vi "PLF.vi"(5 "ActivateAIView":bool, 9 "curr_pos":dbl=50.0 min=50.0 max=150.0, 10 "Y":refnum<data-value>, 11 "K":refnum<data-value>) -> (3 "This VI":refnum<vi>)   [LabVIEW 2019]
uses:
  Inputs/Inputs.lvlib
panel:
  in  "обнулить позицию":bool
  in  "pos_offset":dbl=50.0 min=2.0 max=120.0
  in  "зона нечувствительности":dbl
  in  "Q in":dbl format="%#.2f"
  out "Y 2":dbl format="%#.2f"
  out "XY Graph":cluster{"SP_massiv":dbl[], "Y_massiv":dbl[]}(graph)
  in  "Y_massiv":dbl[](array[numeric]) format="%#.2f"
  in  "SP_massiv":dbl[](array[numeric]) format="%#.2f"
  in  "derivative time (Td, s)":dbl
  in  "integral time (Ti, s)":dbl
  in  "proportional gain (Kc)":dbl
  in  "output high":dbl
  # "Параметры ПИД Регулятора"
  # "Y"
  # "Настройка Выхода"
  # "Q_max"
  # "Q9"
  # "Q8"
  # "Q7"
  # "Q6"
  # "Q5"
  # "Q4"
  # "Q3"
  # "Q2"
  # "Q1"
  # "Q_min"
  # "X"
  # "Y_min"
  # "Y1"
  # "Y2"
  # "Y3"
  # "Y4"
  # "Y5"
  # "Y6"
  # "Y7"
  # "Y8"
  # "Y9"
  # "Y_max"
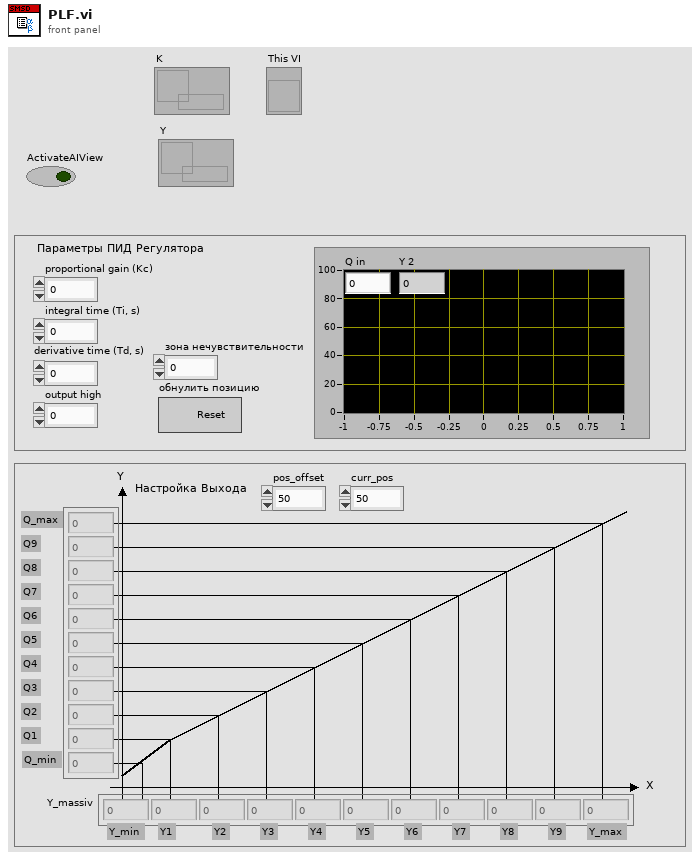
[diagram p1: front panel]
types:
  T1 = enum32{"Invalid", "Standard", "Closed", "Hidden", "Minimized", "Maximized"}
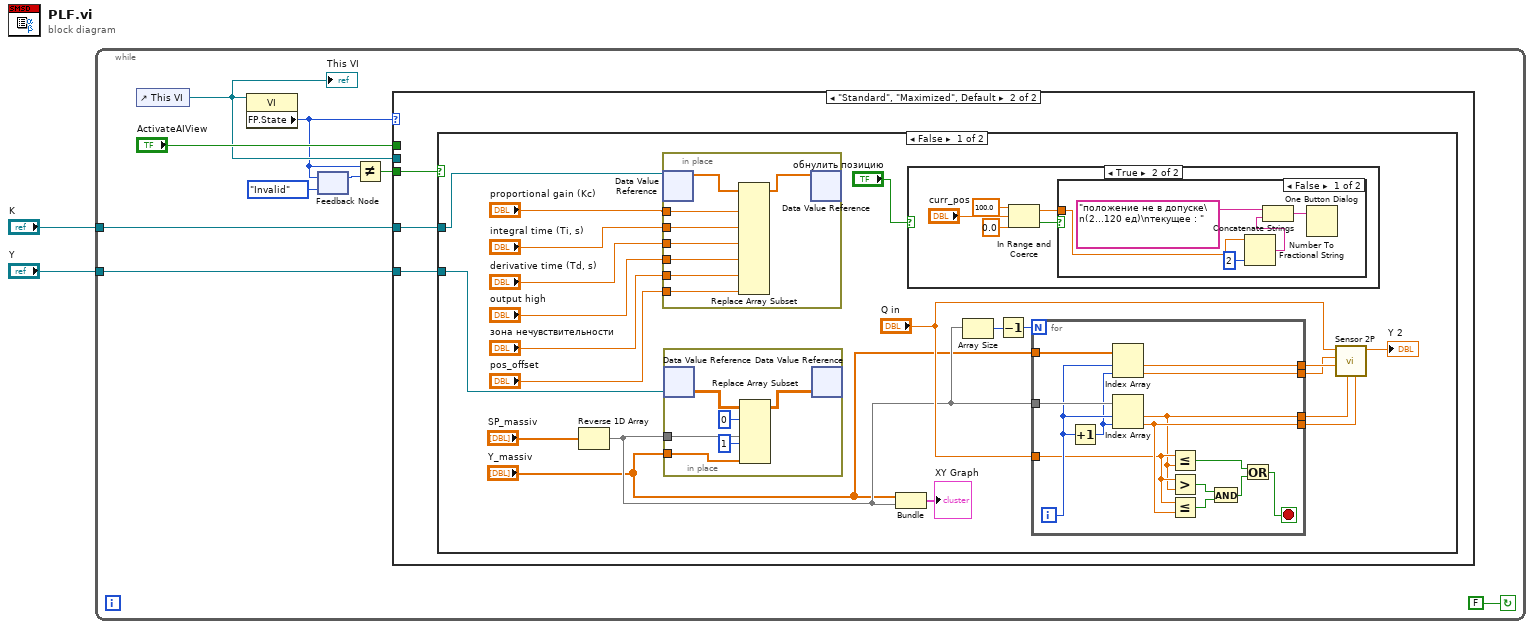
[diagram p0: block diagram]
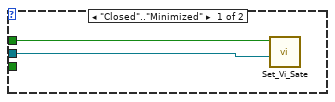
[diagram p2: hidden frame]
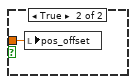
[diagram p4: hidden frame]
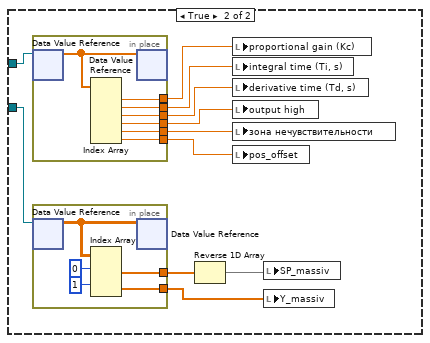
[diagram p5: hidden frame]
diagram:
  n1 = while {
    tunnel: "K" -> [w4]
    tunnel: "Y" -> [w3]
    stop <- FALSE continue-if-true
    n2 = control-ref of="This VI"() -> (w10:refnum<vi>)
    "This VI" <- w10
    n3 = property class="VI"(reference=w10) -> ("FP.State"=w8:T1)  [unwired: 1 in, 2 out]
    n4 = feedback #1(T1."Invalid" ("FP.State")) -> (w9:T1)
    n5 = feedback-in #1(w8) -> ()
    n6 = Not Equal?(x=w8, y=w9) -> (x != y?=w7:bool)
    n7 = case shown="\"Standard\", \"Maximized\", Default" w8 {
      tunnel: "ActivateAIView" -> [w13 _]
      tunnel: w10 -> [w12 _]
      tunnel: w7 -> [_ w16]
      tunnel: w4 -> [_ w15]
      tunnel: w3 -> [_ w14]
      frame "Closed".."Minimized" {
        n8 = call "Set_Vi_Sate.vi"("VI"=w12, "Activate (F)"=w13) -> ()  [unwired: 9 in, 1 out]
      }
      frame "Standard", "Maximized", Default {
        n9 = case shown="False" w16 {
          tunnel: w15 -> [w33 w80]
          tunnel: w14 -> [w32 w79]
          frame False {
            n10 = Reverse 1D Array(array="SP_massiv") -> (reversed array=w22:dbl[])
            n11 = in-place {
              in-place-border: "proportional gain (Kc)" -> [w75]
              in-place-border: "integral time (Ti, s)" -> [w74]
              in-place-border: "derivative time (Td, s)" -> [w73]
              in-place-border: "output high" -> [w71]
              in-place-border: "зона нечувствительности" -> [w70]
              in-place-border: "pos_offset" -> [w69]
              n12 = in-place-dvr #2(w33) -> (w76:dbl[])  [unwired: 1 out]
              n13 = Replace Array Subset(array=w76, new element #1=w75, new element #2=w74, new element #3=w73, new element #4=w71, new element #5=w70, new element #6=w69) -> (w72:dbl[])  [unwired: 6 in]
              n14 = in-place-dvr #2(w72) -> ()  [unwired: 2 out]
            }
            n15 = in-place {
              in-place-border: w22 -> [w66]
              in-place-border: "Y_massiv" -> [w63]
              n16 = in-place-dvr #3(w32) -> (w68:dbl[][])  [unwired: 1 out]
              n17 = Replace Array Subset(array=w68, new element #1=w66, index (row) #1=0 ("index (row)"), new element #2=w63, index (row) #2=1 ("index (row)")) -> (w67:dbl[][])  [unwired: 2 in]
              n18 = in-place-dvr #3(w67) -> ()  [unwired: 2 out]
            }
            n19 = Bundle("Y_massiv"="Y_massiv", w22) -> (→"XY Graph":cluster{"Y_massiv":dbl[], dbl[]})  [unwired: 1 in]
            n20 = case shown="True" "обнулить позицию" {
              frame False {
              }
              frame True {
                n21 = In Range and Coerce(upper limit=100.0, x="curr_pos", lower limit=0.0) -> (coerced(x)=w38:dbl, In Range?=w39:bool)
                n22 = case shown="False" w39 {
                  tunnel: w38 -> [w44 w48]
                  frame False {
                    n23 = Number To Fractional String(number=w44, precision (6)=i16 2) -> (F-format string=w43:string)  [unwired: 2 in]
                    n24 = Concatenate Strings("положение не в допуске\n(2...120 ед)\nтекущее : " ("string"), w43) -> (w47:string)
                    n25 = One Button Dialog(message=w47) -> ()  [unwired: 1 in, 1 out]
                  }
                  frame True {
                    n26 = local write "pos_offset"(w48) -> ()
                  }
                }
              }
            }
            n27 = Array Size(array=w22) -> (size(s)=w24:i32)
            n28 = Decrement(x=w24) -> (x-1=w23:i32)
            n29 = for {
              N: w23 -> [_]
              tunnel: w22 -> [w62]
              tunnel: "Q in" -> [w53]
              tunnel: [w52] -> w27
              tunnel: [w59] -> w28
              tunnel: "Y_massiv" -> [w56]
              tunnel: [w55] -> w26
              tunnel: [w54] -> w25
              i -> [w58]
              stop <- w49 stop-if-true
              n30 = Increment(x=w58) -> (x+1=w57:i32)
              n31 = Index Array(array=w56, index #1=w58, index #2=w57) -> (element #1=w55:dbl, element #2=w54:dbl)
              n32 = Index Array(array=w62, index #1=w58, index #2=w57) -> (element #1=w52:dbl, element #2=w59:dbl)
              n33 = Less Or Equal?(x=w53, y=w52) -> (x <= y?=w50:bool)
              n34 = Greater?(x=w53, y=w52) -> (0:w61:bool)
              n35 = Less Or Equal?(x=w53, y=w59) -> (x <= y?=w60:bool)
              n36 = And(x=w61, y=w60) -> (x .and. y?=w51:bool)
              n37 = Or(x=w50, y=w51) -> (x .or. y?=w49:bool)
            }
            n38 = call "Sensor 2P.vi"("Xmax"=w28, "Xmin"=w27, "Ymin"=w26, "Ymax"=w25, "X"="Q in") -> ("Y"=→"Y 2":dbl)  [unwired: 6 in]
          }
          frame True {
            n39 = in-place {
              in-place-border: [w98] -> w86
              in-place-border: [w97] -> w85
              in-place-border: [w96] -> w84
              in-place-border: [w95] -> w83
              in-place-border: [w94] -> w78
              in-place-border: [w93] -> w77
              n40 = in-place-dvr #4(w80) -> (w99:dbl[])  [unwired: 1 out]
              n41 = Index Array(array=w99) -> (element #1=w98:dbl, element #2=w97:dbl, element #3=w96:dbl, element #4=w95:dbl, element #5=w94:dbl, element #6=w93:dbl)  [unwired: 6 in]
              n42 = in-place-dvr #4(w99) -> ()  [unwired: 2 out]
            }
            n43 = in-place {
              in-place-border: [w91] -> w82
              in-place-border: [w90] -> w81
              n44 = in-place-dvr #5(w79) -> (w92:dbl[][])  [unwired: 1 out]
              n45 = Index Array(array=w92, index (row) #1=0 ("index (row)"), index (row) #2=1 ("index (row)")) -> (element #1=w91:dbl[], element #2=w90:dbl[])  [unwired: 2 in]
              n46 = in-place-dvr #5(w92) -> ()  [unwired: 2 out]
            }
            n47 = Reverse 1D Array(array=w82) -> (reversed array=w87:dbl[])
            n48 = local write "proportional gain (Kc)"(w86) -> ()
            n49 = local write "integral time (Ti, s)"(w85) -> ()
            n50 = local write "derivative time (Td, s)"(w84) -> ()
            n51 = local write "output high"(w83) -> ()
            n52 = local write "зона нечувствительности"(w78) -> ()
            n53 = local write "pos_offset"(w77) -> ()
            n54 = local write "SP_massiv"(w87) -> ()
            n55 = local write "Y_massiv"(w81) -> ()
          }
        }
      }
    }
  }
